vi "System Monitor.vi"(8 "error in (no error)":errorcluster) -> (0 "error out":errorcluster)   [LabVIEW 2024]
doc: "Dialog for selecting user specified settings."
uses:
  <vilib>/nisyscfg/Close (Resources).vi
  <vilib>/nisyscfg/Close (Filter).vi
  <vilib>/nisyscfg/Close (System).vi
  <vilib>/nisyscfg/nisyscfg.lvlib
  <resource>/objmgr/niflexrioatomicsae.rc
panel:
  out "output cluster":T1 {"Temp Readings (C)" format="%#_4g"; "Fan Readings (rpm)" format="%_4f"; "Volt Nominal (V)" format="%#_3g"; "Volt Readings (V)" format="%#_3g"; "Module Temp (C)" format="%#_4g"}
  in  "Close Button":bool
  # "Non visible portion of dialog (needed for connector pane)."
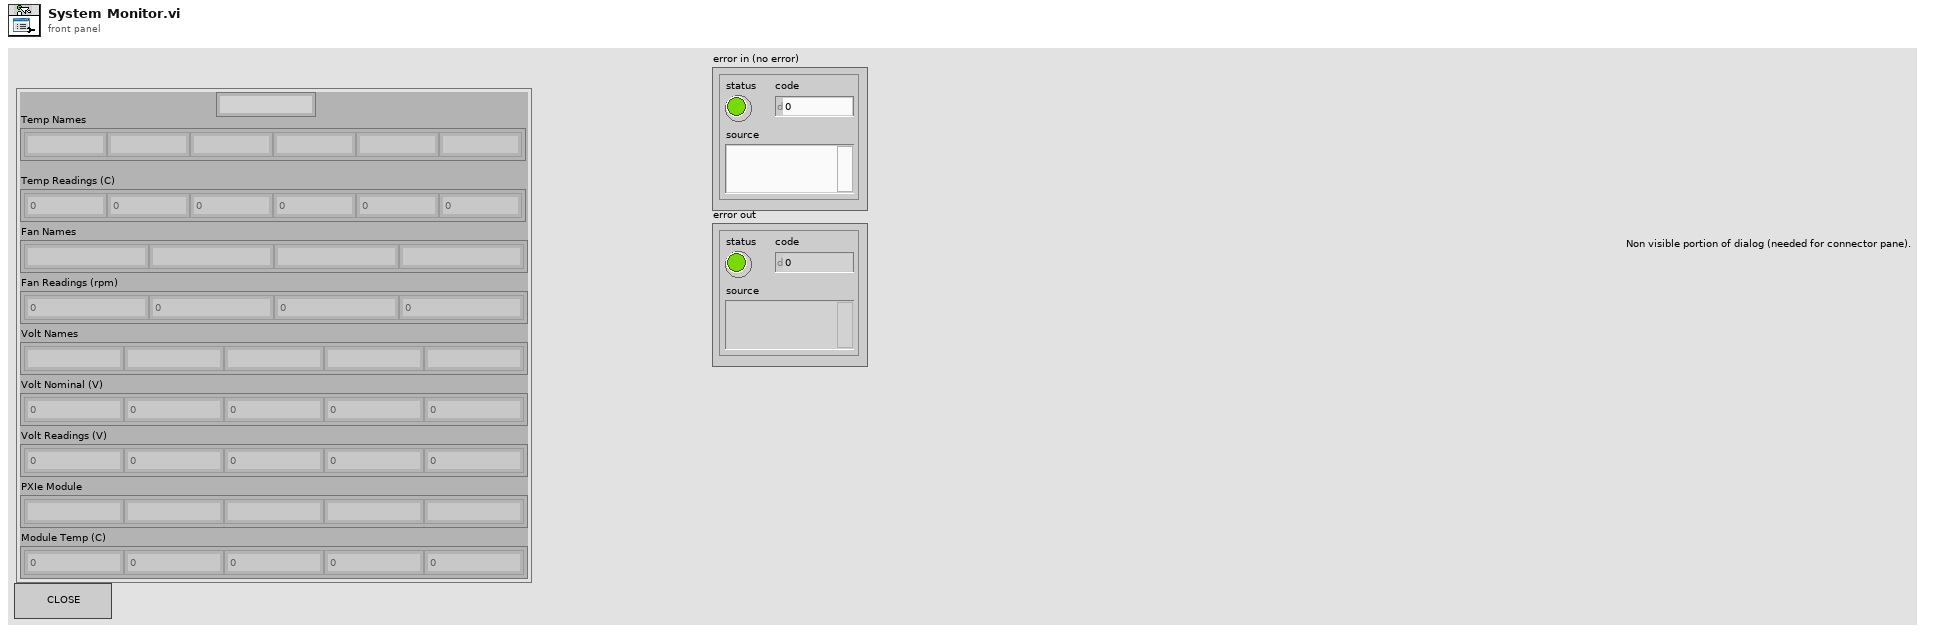
[diagram p1: front panel]
types:
  T1 = cluster{string, "Temp Names":string[], "Temp Readings (C)":dbl[], "Fan Names":string[], "Fan Readings (rpm)":u32[], "Volt Names":string[], "Volt Nominal (V)":dbl[], "Volt Readings (V)":dbl[], "PXIe Module":string[], "Module Temp (C)":dbl[]}
  T2 = cluster{string, "TempNames":string[], "TempReadings":dbl[], "FanNames":string[], "FanReadings":u32[], "VoltNames":string[], "VoltNominal":dbl[], "VoltReadings":dbl[], string[], dbl[]}
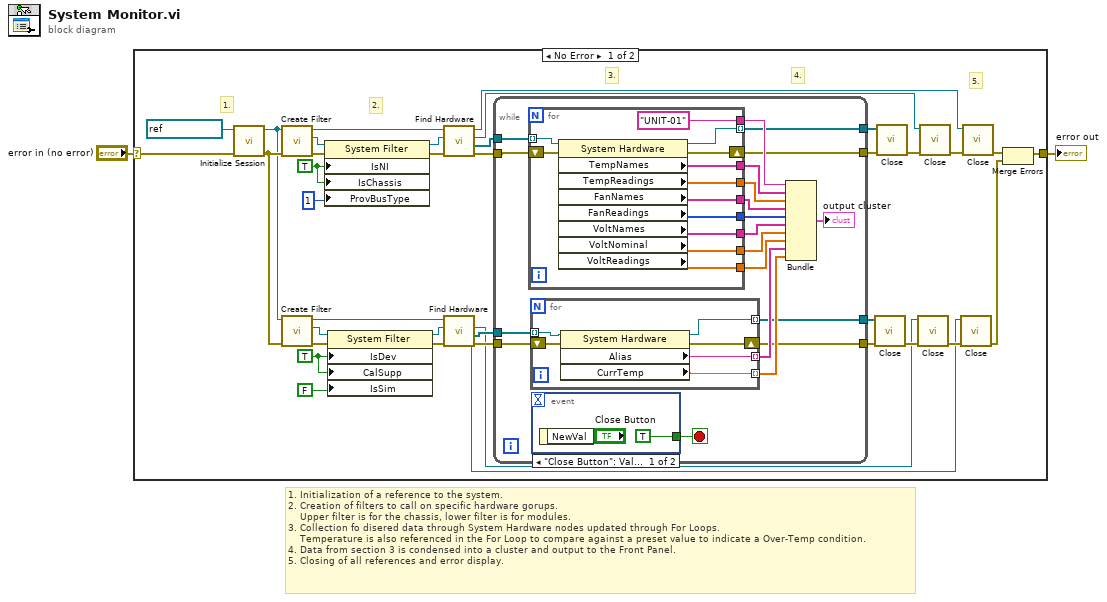
[diagram p0: block diagram]
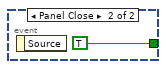
[diagram p2: hidden frame]
diagram:
  # "1. Initialization of a reference to the system.\n2. Creation of filters to call on specific hardware gorups. \n    Upper filter is for the chassis, lower filter is for modules.\n3. Collection fo disered data through System Hardware nodes updated through For Loops. \n    Temperature is also referenced in the For Loop to compare against a preset value to indicate a Over-Temp condition.\n4. Data from section 3 is condensed into a cluster and output to the Front Panel. \n5. Closing of all references and error display."
  n1 = case shown="No Error" "error in (no error)" {
    selector: "error in (no error)" -> [w22 w80]
    tunnel: [w3 w80] -> w2
    frame No Error {
      w25 = TRUE
      w39 = TRUE
      # "4."
      # "3."
      # "5."
      # "2."
      # "1."
      n2 = call <vilib>:"Initialize Session.vi"("error in (no error)"=w22, "Target (localhost)"=refnum<k21> "localhost" ("System Configuration")) -> ("error out"=w32:errorcluster, "Session out"=w31:refnum<k21>)  [unwired: 8 in]
      n3 = call <vilib>:"Create Filter.vi"("error in (no error)"=w32, "Session in"=w31) -> ("error out"=w35:errorcluster, "Filter out"=w23:refnum<k20>, "Session out"=w34:refnum<k21>)  [unwired: 7 in]
      n4 = call <vilib>:"Create Filter.vi"("error in (no error)"=w32, "Session in"=w31) -> ("error out"=w29:errorcluster, "Filter out"=w27:refnum<k20>, "Session out"=w30:refnum<k21>)  [unwired: 7 in]
      n5 = property class="System Filter"(reference=w23, error in=w35, "IsNI"=w39, "IsChassis"=w39, "ProvBusType"=u32 1) -> (reference out=w38:refnum<k20>, error out=w33:errorcluster)
      n6 = property class="System Filter"(reference=w27, error in=w29, "IsDev"=w25, "CalSupp"=w25, "IsSim"=FALSE) -> (reference out=w26:refnum<k20>, error out=w28:errorcluster)
      n7 = call <vilib>:"Find Hardware.vi"("error in (no error)"=w33, "Filter in"=w38, "Session in"=w34) -> ("error out"=w21:errorcluster, "Resources out"=w18:refnum<k20>[], "Filter out"=w12:refnum<k20>, "Session out"=w13:refnum<k21>)  [unwired: 5 in]
      n8 = call <vilib>:"Find Hardware.vi"("error in (no error)"=w28, "Filter in"=w26, "Session in"=w30) -> ("error out"=w20:errorcluster, "Resources out"=w19:refnum<k20>[], "Filter out"=w7:refnum<k20>, "Session out"=w6:refnum<k21>)  [unwired: 5 in]
      n9 = while {
        tunnel: w18 -> [w47]
        tunnel: w21 -> [w46]
        tunnel: w19 -> [w45]
        tunnel: w20 -> [w44]
        tunnel: [w43] -> w9
        tunnel: [w42] -> w8
        tunnel: [w41] -> w10
        tunnel: [w40] -> w11
        stop <- w59 stop-if-true
        n10 = for {
          tunnel: w47 -> [w77] mode=indexing
          shift-right: [w75] -> w40
          shift-left: w46 -> [w76]
          tunnel: [w67] -> w41 mode=indexing
          tunnel: [w74] -> w58
          tunnel: [w73] -> w57
          tunnel: [w72] -> w56
          tunnel: [w71] -> w55
          tunnel: [w70] -> w54
          tunnel: [w66] -> w53
          tunnel: [w69] -> w52
          tunnel: ["UNIT-01"] -> w51
          n11 = property class="System Hardware"(reference=w77, error in=w76) -> (reference out=w67:refnum<k20>, error out=w75:errorcluster, "TempNames"=w69:string[], "TempReadings"=w66:dbl[], "FanNames"=w70:string[], "FanReadings"=w71:u32[], "VoltNames"=w72:string[], "VoltNominal"=w73:dbl[], "VoltReadings"=w74:dbl[])
        }
        n12 = for {
          shift-right: [w64] -> w42
          shift-left: w44 -> [w65]
          tunnel: [w63] -> w50 mode=indexing
          tunnel: [w60] -> w49 mode=indexing
          tunnel: [w62] -> w43 mode=indexing
          tunnel: w45 -> [w61] mode=indexing
          n13 = property class="System Hardware"(reference=w61, error in=w65) -> (reference out=w62:refnum<k20>, error out=w64:errorcluster, "Alias"=w63:string, "CurrTemp"=w60:dbl)
        }
        n14 = event shown="[0] \"Close Button\": Value Change" {
          selector: _ -> [_ _]
          dyn-events: _ -> [_ _]
          timeout: _ -> [_ _]
          tunnel: [TRUE TRUE] -> w59
          event "Close Button": Value Change {
            n15 = event-data() -> ()  [unwired: 1 in, 1 out]
          }
          event Panel Close {
            n16 = event-data() -> ()  [unwired: 1 in, 1 out]
          }
        }
        n17 = Bundle(w51, "TempNames"=w52, "TempReadings"=w53, "FanNames"=w54, "FanReadings"=w55, "VoltNames"=w56, "VoltNominal"=w57, "VoltReadings"=w58, w50, w49) -> (→"output cluster":T2)  [unwired: 1 in]
      }
      n18 = call-poly <vilib>:"Close.vi"("error in (no error)"=w8, "Resources in"=w9) -> ("error out"=w15:errorcluster)  [unwired: 9 in]
      n19 = call-poly <vilib>:"Close.vi"("error in (no error)"=w11, "Resources in"=w10) -> ("error out"=w17:errorcluster)  [unwired: 9 in]
      n20 = call-poly <vilib>:"Close.vi"("error in (no error)"=w15, "Filter in"=w7) -> ("error out"=w14:errorcluster)  [unwired: 9 in]
      n21 = call-poly <vilib>:"Close.vi"("error in (no error)"=w17, "Filter in"=w12) -> ("error out"=w16:errorcluster)  [unwired: 9 in]
      n22 = call-poly <vilib>:"Close.vi"("error in (no error)"=w14, "Session in"=w6) -> ("error out"=w4:errorcluster)  [unwired: 9 in]
      n23 = call-poly <vilib>:"Close.vi"("error in (no error)"=w16, "Session in"=w13) -> ("error out"=w5:errorcluster)  [unwired: 9 in]
      n24 = Merge Errors(w5, w4) -> (w3:errorcluster)
    }
    frame Error {
    }
  }
  "error out" <- w2
